vi "Write Pressure to Logfile.vi"(8 "error in (no error)":errorcluster, 9 "Manifold Pressure (Pa)":dbl, 10 "Tube Pressure (Pa)":dbl, 11 "tdms file":refnum<k34>) -> (0 "error out":errorcluster, 3 "tdms file out":refnum<k34>)   [LabVIEW 2018]
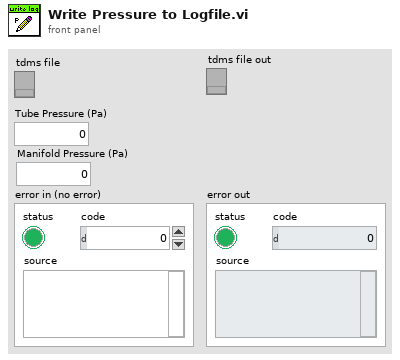
[diagram p1: front panel]
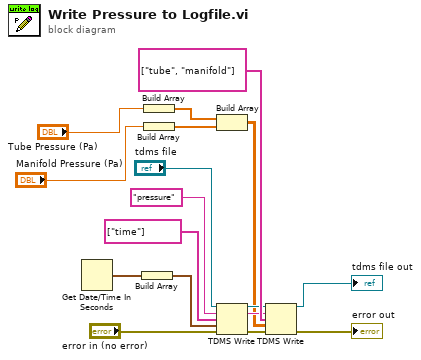
[diagram p0: block diagram]
diagram:
  n1 = Get Date/Time In Seconds() -> (seconds since 1Jan1904=w15:timestamp)
  n2 = Build Array(w15) -> (w14:timestamp[])
  n3 = Build Array("Tube Pressure (Pa)") -> (w9:dbl[])
  n4 = Build Array("Manifold Pressure (Pa)") -> (w8:dbl[])
  n5 = Build Array(w9, w8) -> (w7:dbl[][])
  n6 = TDMS Write(0:"tdms file", 5:"pressure" ("group name in (Untitled)"), 7:string[] ["time"] ("channel name(s) in (Untitled)"), 9:w14, 11:"error in (no error)") -> (4:w13:refnum<k34>, 6:w12:string, 15:w16:errorcluster)  [unwired: 1 in, 1 out]
  n7 = TDMS Write(0:w13, 5:w12, 7:string[] ["tube", "manifold"] ("channel name(s) in (Untitled)"), 9:w7, 11:w16) -> (4:→"tdms file out":refnum<k34>, 15:→"error out":errorcluster)  [unwired: 1 in, 2 out]
